vi "AddDefaultBDModules.vi"(8 "error in":errorcluster, 11 "PythonConverter_BD in":refnum<class "PyConvBD.lvclass">) -> (0 "error out":errorcluster, 3 "PythonConverter_BD out":refnum<class "PyConvBD.lvclass">)   [LabVIEW 2014, in "Raspberry Pi Compatible Compiler for LabVIEW.lvlib" / "PyConvBD.lvclass"]
uses:
  PyConvBD.lvclass
  PyConvBD.lvclass/PyConvBD.ctl
panel:
  in  "BD modules":T1(array[cluster])=[{"Python module"="pyVI.BD.lvNodes", "Python module  name"="lvNode"}, {"Python module"="pyVI.VI.lvDataTypes", "Python module  name"="lvDT"}, {"Python module"="pyVI.BD.lvStructures", "Python module  name"="lvStruct"}, {"Python module"="concurrent.futures", "Python module  name"="futures"}]
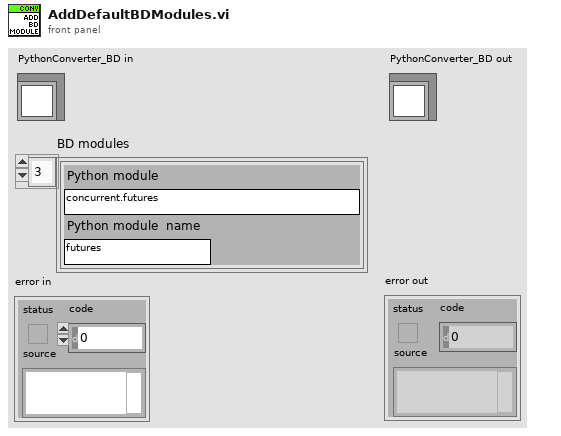
[diagram p1: front panel]
types:
  T1 = cluster{"Python module":string, "Python module  name":string}[]
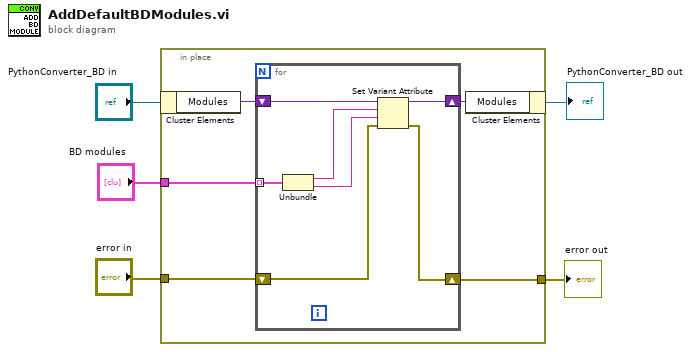
[diagram p0: block diagram]
diagram:
  n1 = in-place {
    in-place-border: "error in" -> [w8]
    in-place-border: [w7] -> w1
    in-place-border: "BD modules" -> [w6]
    n2 = in-place-cluster #1("PythonConverter_BD in") -> ("Modules"=w10:variant)
    n3 = for {
      shift-right: [w16] -> w9
      shift-left: w10 -> [w17]
      shift-right: [w14] -> w7
      shift-left: w8 -> [w15]
      tunnel: w6 -> [w13] mode=indexing
      n4 = Unbundle(w13) -> ("Python module"=w12:string, "Python module  name"=w11:string)
      n5 = Set Variant Attribute(Variant=w17, name=w12, value=w11, error in=w15) -> (Variant out=w16:variant, error out=w14:errorcluster)  [unwired: 1 out]
    }
    n6 = in-place-cluster #1("Modules"=w9) -> (→"PythonConverter_BD out":refnum<class "PyConvBD.lvclass">)
  }
  "error out" <- w1
